vi "UDP - 副本.vi"() -> ()   [LabVIEW 2010]
panel:
  in  "接收本地端口":u16
  in  "发送本地端口":u16
  in  "远程主机IP":string
  in  "发送远程端口":u16
  out "接收数据":string
  in  "发送数据":string
  in  "发送":bool
  in  "关闭":bool
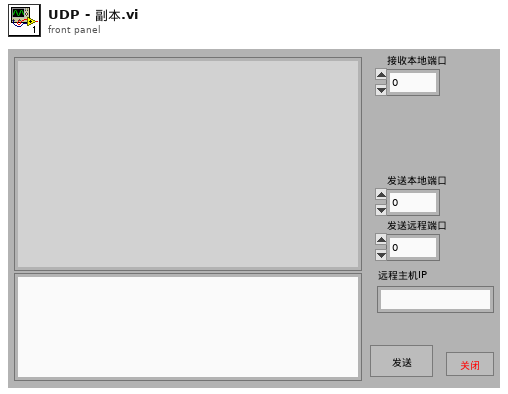
[diagram p1: front panel]
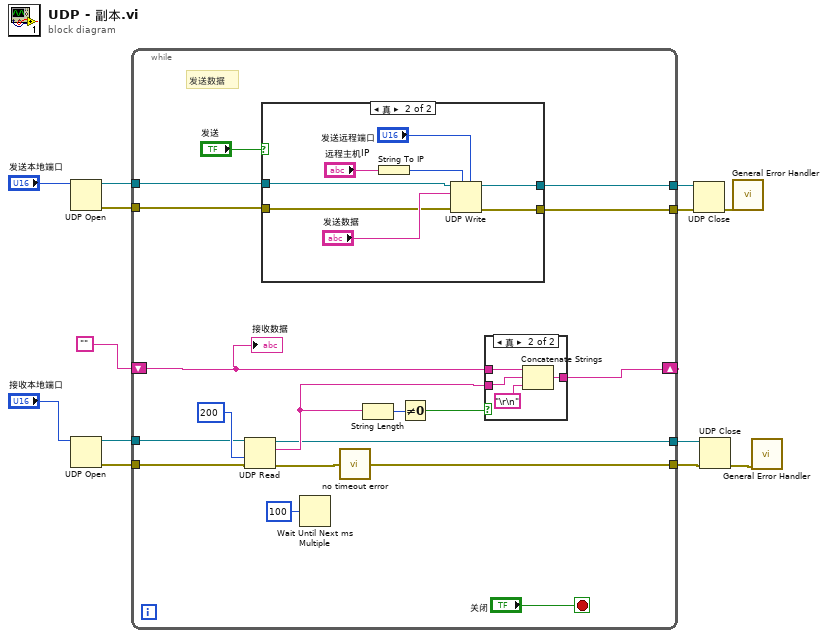
[diagram p0: block diagram]
diagram:
  n1 = UDP Open(11:"发送本地端口") -> (port=w8:refnum<k16>, 0:w7:errorcluster)  [unwired: 4 in, 1 out]
  n2 = UDP Open(11:"接收本地端口") -> (port=w10:refnum<k16>, 0:w9:errorcluster)  [unwired: 4 in, 1 out]
  n3 = while {
    shift-right: [w22] -> _
    shift-left: "" -> [w23]
    tunnel: w10 -> [w21]
    tunnel: w9 -> [w20]
    tunnel: w8 -> [w14]
    tunnel: w7 -> [w19]
    tunnel: [w18] -> w4
    tunnel: [w17] -> w3
    tunnel: [w16] -> w2
    tunnel: [w15] -> w1
    stop <- "关闭" stop-if-true
    # "发送数据"
    n4 = UDP Read(connection ID=w21, timeout ms (25000)=200, 8:w20) -> (data out=w26:string, error out=w24:errorcluster, 3:w16:refnum<k16>)  [unwired: 1 in, 2 out]
    n5 = case shown="真" "发送" {
      tunnel: w19 -> [w38 w43]
      tunnel: [w37 w42] -> w18
      tunnel: [w38 w41] -> w17
      tunnel: w14 -> [w37 w39]
      frame False {
      }
      frame True {
        n6 = String To IP(1:"远程主机IP") -> (0:w45:u32)
        n7 = UDP Write(address=w45, port or service name="发送远程端口", connection ID=w39, data in="发送数据", 8:w43) -> (error out=w41:errorcluster, 3:w42:refnum<k16>)  [unwired: 1 in]
      }
    }
    n8 = Wait Until Next ms Multiple(millisecond multiple=u32 100) -> ()  [unwired: 1 out]
    n9 = call "no timeout error.vi"("error in (no error)"=w24) -> ("error out"=w15:errorcluster)
    n10 = String Length(string=w26) -> (length=w28:i32)
    n11 = Not Equal To 0?(x=w28) -> (x != 0?=w27:bool)
    n12 = case shown="真" w27 {
      tunnel: w23 -> [w32 w36]
      tunnel: w26 -> [_ w34]
      tunnel: [w32 w35] -> w22
      frame False {
      }
      frame True {
        n13 = Concatenate Strings(w36, w34, "\r\n" ("Substring")) -> (w35:string)
      }
    }
    "接收数据" <- w23
  }
  n14 = UDP Close(connection ID=w4, 8:w3) -> (error out=w6:errorcluster)  [unwired: 1 out]
  n15 = UDP Close(connection ID=w2, 8:w1) -> (error out=w5:errorcluster)  [unwired: 1 out]
  n16 = call <vilib>:"General Error Handler.vi"("error in (no error)"=w6) -> ()  [unwired: 10 in, 5 out]
  n17 = call <vilib>:"General Error Handler.vi"("error in (no error)"=w5) -> ()  [unwired: 10 in, 5 out]
